vi "SecondaryJoystickAcquire.vi"(8 "Rotation Joystick Deadband %":dbl, 11 "XY Joystick Deadband %":dbl) -> (0 "Secondary Joystick Buttons":bool[](array[boolean]), 3 "Secondary Joystick Values":dbl[](array[numeric]))   [LabVIEW 2018]
uses:
  <vilib>/Rock Robotics/WPI/Utilities/WPI_GetSetVariantRefNum.vi
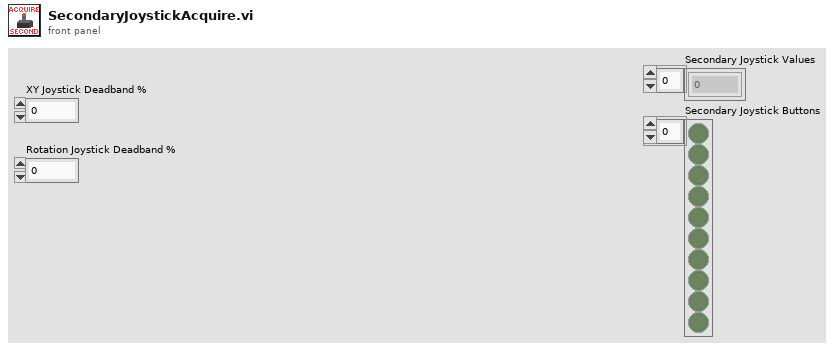
[diagram p1: front panel]
types:
  T1 = typedef "WPI_JoystickDevRef.ctl" = cluster{"Device":T2}
  T2 = typedef "WPI_JoystickDeviceEnum.ctl" = enum16{"USB 0", "USB 1", "USB 2", "USB 3", "USB 4", "USB 5"}
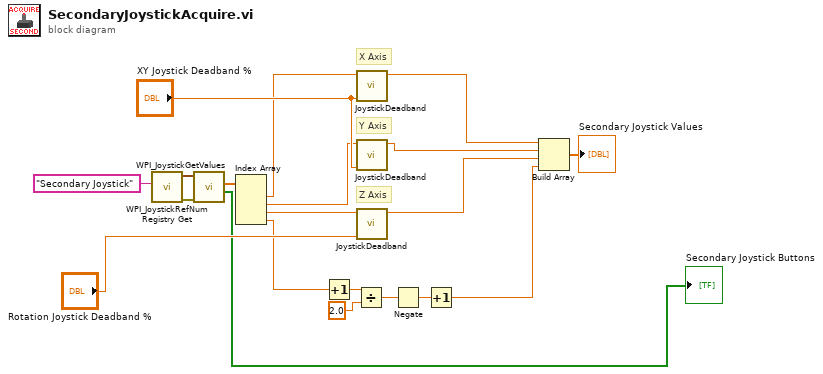
[diagram p0: block diagram]
diagram:
  # "Z Axis"
  # "Y Axis"
  # "X Axis"
  n1 = call <vilib>:"WPI_JoystickRefNum Registry Get.vi"("refnum name"="Secondary Joystick") -> ("error out"=w20:errorcluster, "JoystickDevRef"=w19:T1)  [unwired: 9 in]
  n2 = call <vilib>:"WPI_JoystickGetValues.vi"("error in (no error)"=w20, "JoystickDevRef"=w19) -> ("Buttons"=→"Secondary Joystick Buttons":bool[], "Axes"=w16:dbl[])  [unwired: 5 in, 3 out]
  n3 = Index Array(array=w16) -> (element #1=w15:dbl, element #2=w14:dbl, element #3=w13:dbl, element #4=w9:dbl)  [unwired: 4 in]
  n4 = Increment(x=w9) -> (x+1=w10:dbl)
  n5 = Divide(x=w10, y=2.0) -> (x/y=w8:dbl)
  n6 = call "JoystickDeadband.vi"("Deadband %"="XY Joystick Deadband %", "Joystick Value"=w15) -> ("Joystick Value"=w3:dbl)  [unwired: 9 in]
  n7 = call "JoystickDeadband.vi"("Deadband %"="XY Joystick Deadband %", "Joystick Value"=w14) -> ("Joystick Value"=w4:dbl)  [unwired: 9 in]
  n8 = call "JoystickDeadband.vi"("Deadband %"="Rotation Joystick Deadband %", "Joystick Value"=w13) -> ("Joystick Value"=w5:dbl)  [unwired: 9 in]
  n9 = Negate(x=w8) -> (-x=w7:dbl)
  n10 = Increment(x=w7) -> (x+1=w6:dbl)
  n11 = Build Array(w3, w4, w5, w6) -> (→"Secondary Joystick Values":dbl[])
